vi "WriteConfgInpt_KtypeTC.vi"(8 "error in (no error)":errorcluster, 10 "Port Number":u16=2000, 11 "IP Address":string="192.168.12.200") -> (0 "error out":errorcluster, 3 "Output Reading":string="W01\r\n")   [LabVIEW 2013, in "ovenCtrl.lvlib"]
uses:
  ovenCtrl.lvlib
panel:
  # "Inputs"
  # "Outputs"
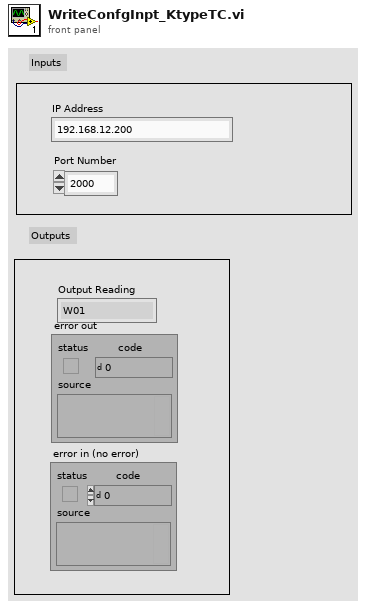
[diagram p1: front panel]
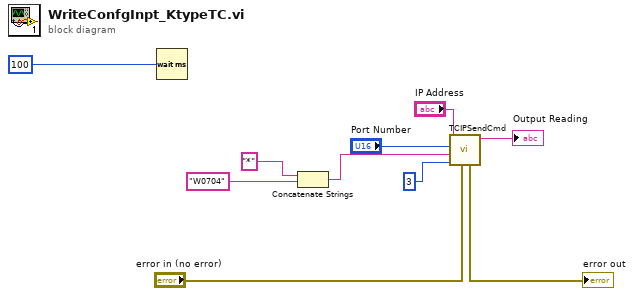
[diagram p0: block diagram]
diagram:
  n1 = Wait (ms)(milliseconds to wait=u32 100) -> ()  [unwired: 1 out]
  n2 = Concatenate Strings("*" ("string"), "W0704" ("string")) -> (w4:string)
  n3 = call "TCIPSendCmd.vi"("error in (no error)"="error in (no error)", "bytes to read"=3, "Command"=w4, "Port Number"="Port Number", "IP Address"="IP Address") -> ("Output Reading"=→"Output Reading":string, "error out"=→"error out":errorcluster)  [unwired: 5 in]
